vi "onDestroyHttpSession.vi"(8 "error in (no error)":errorcluster, 11 "advanced-http-client in":refnum<class "advanced-http-client.lvclass">) -> (0 "error out":errorcluster, 3 "advanced-http-client out":refnum<class "advanced-http-client.lvclass">)   [LabVIEW 2020, in "HttpClient.NiAdvanced.lvlib" / "advanced-http-client.lvclass"]
uses:
  advanced-http-client.lvclass
  advanced-http-client.lvclass/advanced-http-client.ctl
  <vilib>/NI/Advanced HTTP Client/Session.lvclass
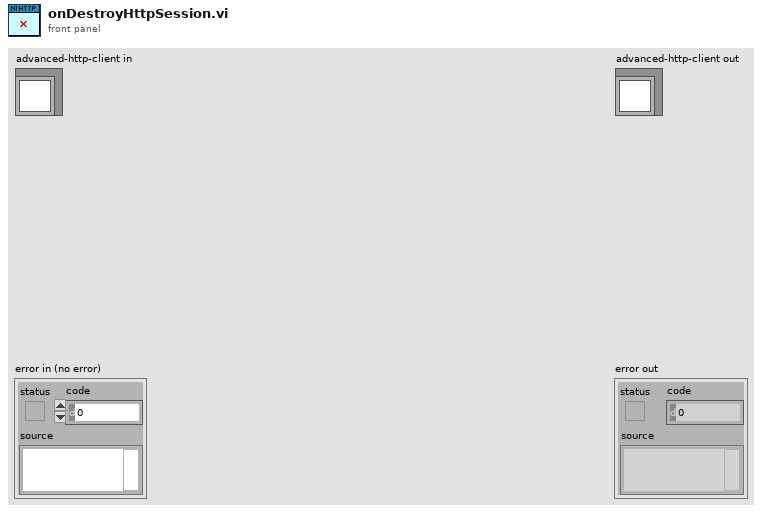
[diagram p1: front panel]
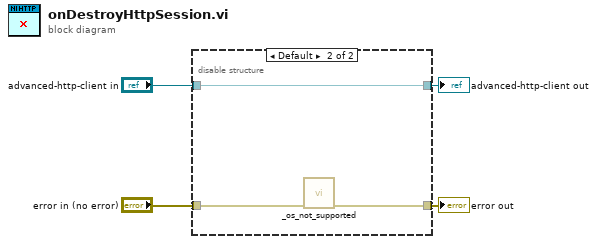
[diagram p0: block diagram]
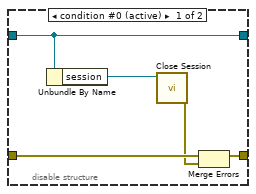
[diagram p2: hidden frame]
diagram:
  n1 = disable-structure shown="Default" {
    disable-tunnel: "advanced-http-client in" -> [w5 w12]
    disable-tunnel: [w9 w10] -> w3
    disable-tunnel: "error in (no error)" -> [w8 w11]
    disable-tunnel: [w5 w12] -> w1
    frame condition #0 (active) {
      n2 = Unbundle By Name(w5) -> ("session"=w7:refnum<class "Session.lvclass">)
      n3 = call <vilib>:"Close Session.vi"("session"=w7) -> ("error out"=w6:errorcluster)  [unwired: 10 in]
      n4 = Merge Errors(w8, w6) -> (w9:errorcluster)
    }
    frame condition #1 {
      n5 = call "_os_not_supported.vi"("error in (no error)"=w11) -> ("error out"=w10:errorcluster)  [unwired: 9 in, 1 out]
    }
  }
  "error out" <- w3
  "advanced-http-client out" <- w1
